vi "Main.vi"() -> ()   [LabVIEW 2019]
panel:
  in  "Warning sound":bool
  in  "Bypass the FMag status":bool
  out "Beam Permit":bool
  in  "Force ON Beam permit":bool
  in  "Force OFF Beam permit":bool
  out "Beam permit status":string
  out "Warning play time":u32
  out "TCP":bool
  in  "Exit VI":bool
  out "Fmag Low Current attemps":i32
  out "Error status":T1(ring)
  out "FMag monitor":u8(slide) scale=0.0..25.0
  out "chart_temp 2":waveform(dbl)[](graph)=[{"t0"=timestamp(3772890114.31303 s since 1904-01-01), "dt"=1.0, "Y"=[0.8687935985565186]}, {"t0"=timestamp(3772890114.31303 s since 1904-01-01), "dt"=1.0, "Y"=[86.87935985565186]}, {"t0"=timestamp(3772890114.31303 s since 1904-01-01), "dt"=1.0, "Y"=[30.48853325313992]}, {"t0"=timestamp(3772890114.31303 s since 1904-01-01), "dt"=1.0, "Y"=[303.6385332531399]}] caption="FMag Current"
  out "FMag Current (A)":dbl
  out "error out":errorcluster
  out "Target  Ready":bool
  out "FMag Ready":bool
  # "SpinQuest Beam Permit Signaller"
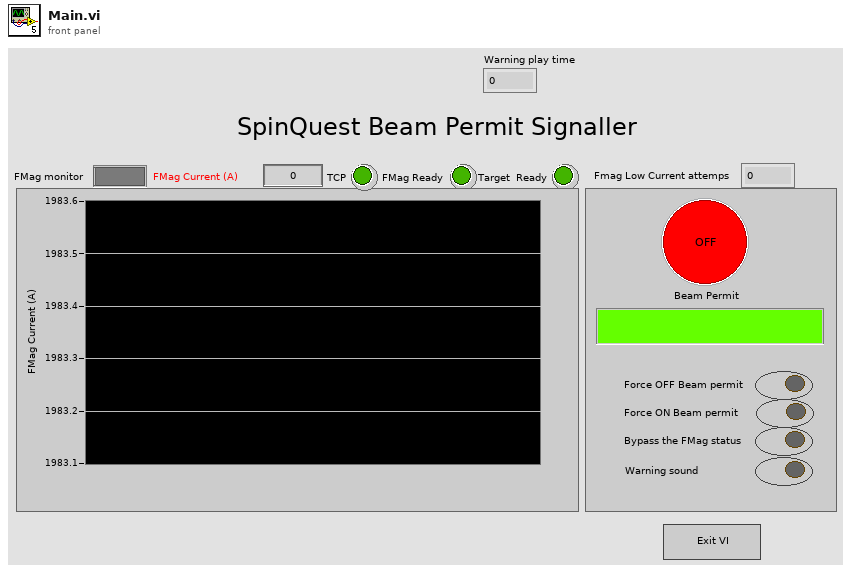
[diagram p1: front panel]
types:
  T1 = enum16{"No Error", "Les than 1800", "Les than 1500", "Les than 200", "Read out Error"}
  T2 = typedef "Sound Output Task ID.ctl" = u32
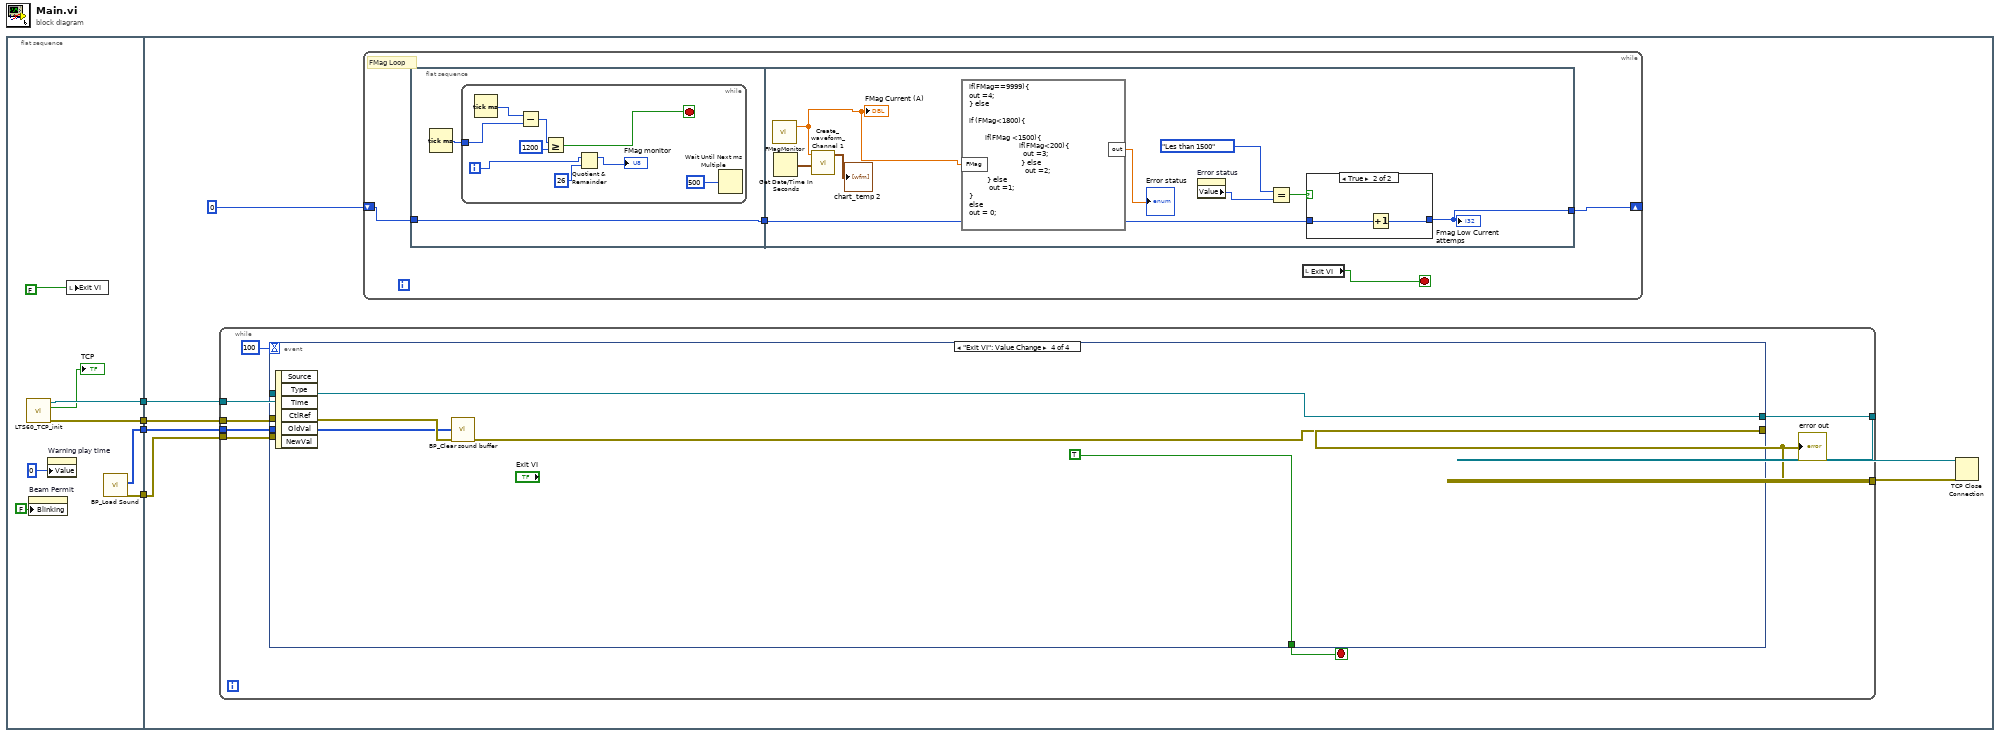
[diagram p0: block diagram]
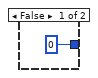
[diagram p2: hidden frame]
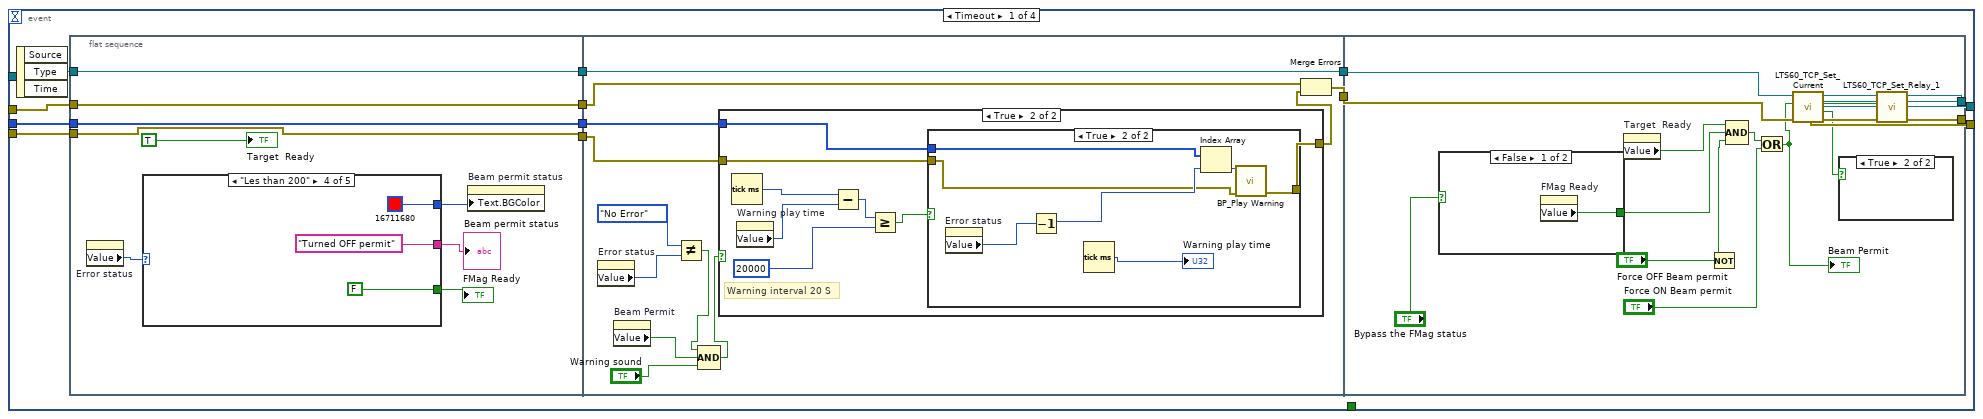
[diagram p3: hidden frame]
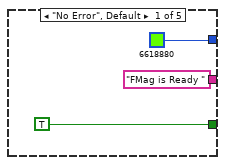
[diagram p4: hidden frame]
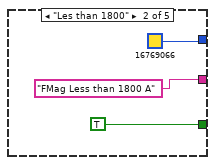
[diagram p5: hidden frame]
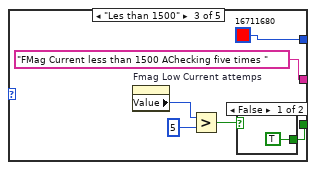
[diagram p6: hidden frame]
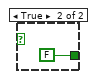
[diagram p7: hidden frame]
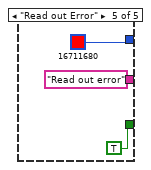
[diagram p8: hidden frame]
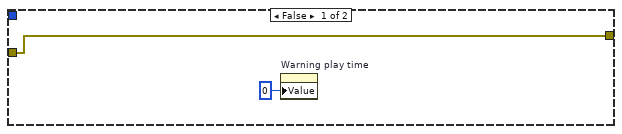
[diagram p9: hidden frame]
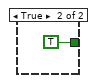
[diagram p12: hidden frame]
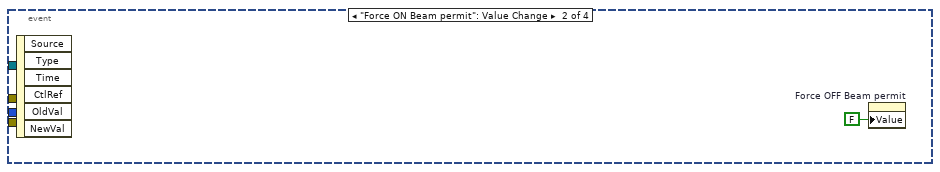
[diagram p13: hidden frame]
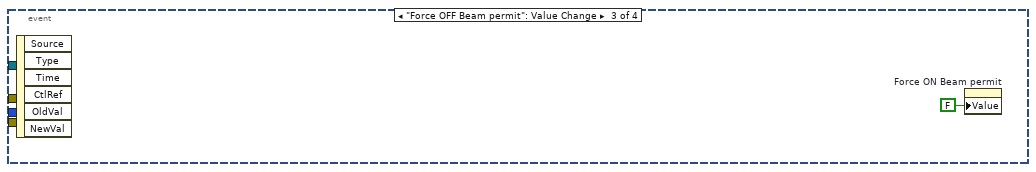
[diagram p14: hidden frame]
diagram:
  n1 = flat-sequence {
    tunnel: [w12] -> w4
    tunnel: [w11] -> w3
    tunnel: [w7] -> w2
    tunnel: [w5] -> w1
    tunnel: w4 -> [w14]
    tunnel: w3 -> [w17]
    tunnel: w2 -> [w15]
    tunnel: w1 -> [w13]
    frame #0 {
      n2 = call "LTS60_TCP_init.vi"() -> ("error out"=w12:errorcluster, "TCP Connected"=→"TCP":bool, "connection ID out"=w11:refnum<k5>)  [unwired: 9 in]
      n3 = property on="Beam Permit" class="Bool (strict)"("Blinking"=FALSE) -> ()  [unwired: 2 in, 2 out]
      n4 = property on="Warning play time" class="DigNum (strict)"("Value"=u32 0 ("Warning play time")) -> ()  [unwired: 2 in, 2 out]
      n5 = local write "Exit VI"(FALSE ("Exit VI")) -> ()
      n6 = call "BP_Load Sound.vi"() -> ("error out"=w5:errorcluster, "Sound Array"=w7:T2[])  [unwired: 9 in, 1 out]
    }
    frame #1 {
      n7 = while {
        tunnel: [w52] -> w18
        tunnel: [w51] -> w19
        tunnel: w14 -> [w50]
        tunnel: w17 -> [w49]
        tunnel: w15 -> [w48]
        tunnel: w13 -> [w47]
        stop <- w54 stop-if-true
        n8 = event shown="[3] \"Exit VI\": Value Change" {
          selector: _ -> [_ _ _ _]
          dyn-events: _ -> [_ _ _ _]
          timeout: 100 -> [_ _ _ _]
          tunnel: [_ _ _ TRUE] -> w54
          tunnel: [w66 _ _ w146] -> w52
          tunnel: [w65 _ _ w149] -> w51
          tunnel: w49 -> [w63 _ _ w149]
          tunnel: w50 -> [w60 _ _ w148]
          tunnel: w48 -> [w58 _ _ w147]
          tunnel: w47 -> [w55 _ _ _]
          event Timeout {
            n9 = event-data() -> ()  [unwired: 1 in, 3 out]
            n10 = flat-sequence {
              tunnel: [w74] -> w64
              tunnel: w63 -> [w74]
              tunnel: [w73] -> w61
              tunnel: w60 -> [w73]
              tunnel: w58 -> [w69]
              tunnel: [w69] -> w57
              tunnel: [w68] -> w56
              tunnel: w55 -> [w68]
              tunnel: w64 -> [w107]
              tunnel: [w107] -> w62
              tunnel: w61 -> [w96]
              tunnel: [w98] -> w59
              tunnel: w57 -> [w104]
              tunnel: w56 -> [w99]
              tunnel: [w137] -> w66
              tunnel: [w136] -> w65
              tunnel: w62 -> [w140]
              tunnel: w59 -> [w134]
              frame #0 {
                n11 = property on="Error status" class="Enum (strict)"() -> ("Value"=w70:T1)  [unwired: 2 in, 2 out]
                n12 = case shown="\"Les than 200\"" w70 {
                  tunnel: [TRUE ("Magnet status") TRUE ("Magnet status") w87 FALSE ("Magnet status") TRUE ("Magnet status")] -> w71
                  tunnel: ["FMag is Ready " ("Beam permit status") "FMag Less than 1800 A" ("Beam permit status") "FMag Current less than 1500 AChecking five times " ("Beam permit status") "Turned OFF permit" ("Beam permit status") "Read out error" ("Beam permit status")] -> w72
                  tunnel: [u32 6618880 ("Text.Text Colors:BG Color") u32 16769066 ("Text.Text Colors:BG Color") u32 16711680 ("Text.Text Colors:BG Color") u32 16711680 ("Text.Text Colors:BG Color") u32 16711680 ("Text.Text Colors:BG Color")] -> w67
                  frame "No Error", Default {
                  }
                  frame "Les than 1800" {
                  }
                  frame "Les than 1500" {
                    n13 = property on="Fmag Low Current attemps" class="DigNum (strict)"() -> ("Value"=w86:i32)  [unwired: 2 in, 2 out]
                    n14 = Greater?(x=w86, y=5) -> (0:w84:bool)
                    n15 = case shown="False" w84 {
                      tunnel: [TRUE ("Magnet status") FALSE ("Magnet status")] -> w87
                      frame False {
                      }
                      frame True {
                      }
                    }
                  }
                  frame "Les than 200" {
                  }
                  frame "Read out Error" {
                  }
                }
                "FMag Ready" <- w71
                "Beam permit status" <- w72
                n16 = property on="Beam permit status" class="Str"("Text.BGColor"=w67) -> ()  [unwired: 2 in, 2 out]
                "Target  Ready" <- TRUE ("Target  status")
              }
              frame #1 {
                n17 = property on="Error status" class="Enum (strict)"() -> ("Value"=w106:T1)  [unwired: 2 in, 2 out]
                n18 = property on="Beam Permit" class="Bool (strict)"() -> ("Value"=w102:bool)  [unwired: 2 in, 2 out]
                n19 = Not Equal?(x=T1."No Error", y=w106) -> (x != y?=w101:bool)
                n20 = Compound Arithmetic op=AND(w101, w102, "Warning sound") -> (w100:bool)
                n21 = case shown="True" w100 {
                  tunnel: w104 -> [_ w112]
                  tunnel: [w108 w111] -> w97
                  tunnel: w99 -> [w108 w110]
                  frame False {
                    n22 = property on="Warning play time" class="DigNum (strict)"("Value"=u32 0 ("Warning play time")) -> ()  [unwired: 2 in, 2 out]
                  }
                  frame True {
                    # "Warning interval 20 S"
                    n23 = Tick Count (ms)() -> (millisecond timer value=w117:u32)
                    n24 = property on="Warning play time" class="DigNum (strict)"() -> ("Value"=w116:u32)  [unwired: 2 in, 2 out]
                    n25 = Subtract(x=w117, y=w116) -> (x-y=w115:u32)
                    n26 = Greater Or Equal?(x=w115, y=u32 20000) -> (x >= y?=w113:bool)
                    n27 = case shown="True" w113 {
                      tunnel: w112 -> [_ w123]
                      tunnel: [w118 w120] -> w111
                      tunnel: w110 -> [w118 w119]
                      frame False {
                      }
                      frame True {
                        n28 = property on="Error status" class="Enum (strict)"() -> ("Value"=w125:T1)  [unwired: 2 in, 2 out]
                        n29 = Decrement(x=w125) -> (x-1=w122:T1)
                        n30 = Tick Count (ms)() -> (millisecond timer value=→"Warning play time":u32)
                        n31 = Index Array(array=w123, index=w122) -> (element=w121:T2)
                        n32 = call "BP_Play Warning.vi"("error in (no error)"=w119, "task ID"=w121) -> ("error out"=w120:errorcluster)  [unwired: 8 in, 1 out]
                      }
                    }
                  }
                }
                n33 = Merge Errors(w96, w97) -> (w98:errorcluster)
              }
              frame #2 {
                n34 = case shown="False" "Bypass the FMag status" {
                  tunnel: [w142 TRUE ("Value")] -> w130
                  frame False {
                    n35 = property on="FMag Ready" class="Bool (strict)"() -> ("Value"=w142:bool)  [unwired: 2 in, 2 out]
                  }
                  frame True {
                  }
                }
                n36 = property on="Target  Ready" class="Bool (strict)"() -> ("Value"=w141:bool)  [unwired: 2 in, 2 out]
                n37 = Not(x="Force OFF Beam permit") -> (.not. x?=w129:bool)
                n38 = Compound Arithmetic op=AND(w141, w130, w129) -> (w132:bool)
                n39 = Or(x=w132, y="Force ON Beam permit") -> (x .or. y?=w127:bool)
                "Beam Permit" <- w127
                n40 = call "LTS60_TCP_Set_Current.vi"("error in (no error)"=w134, "Beam"=w127, "connection ID"=w140) -> ("error out"=w138:errorcluster, "Acknowladged"=w126:bool, "Beam out"=w135:bool, "connection ID out"=w139:refnum<k5>)  [unwired: 5 in]
                n41 = case shown="True" w126 {
                  frame False {
                  }
                  frame True {
                  }
                }
                n42 = call "LTS60_TCP_Set_Relay_1.vi"("error in (no error)"=w138, "Beam"=w135, "connection ID"=w139) -> ("error out"=w137:errorcluster, "connection ID out"=w136:refnum<k5>)  [unwired: 6 in, 1 out]
              }
            }
          }
          event "Force ON Beam permit": Value Change {
            n43 = event-data() -> ()  [unwired: 1 in, 6 out]
            n44 = property on="Force OFF Beam permit" class="Bool (strict)"("Value"=FALSE ("Force OFF Beam permit")) -> ()  [unwired: 2 in, 2 out]
          }
          event "Force OFF Beam permit": Value Change {
            n45 = event-data() -> ()  [unwired: 1 in, 6 out]
            n46 = property on="Force ON Beam permit" class="Bool (strict)"("Value"=FALSE ("Force ON Beam permit")) -> ()  [unwired: 2 in, 2 out]
          }
          event "Exit VI": Value Change {
            n47 = event-data() -> ()  [unwired: 1 in, 6 out]
            n48 = call "BP_Clear sound buffer.vi"("error in (no error)"=w148, "array"=w147) -> ("error out"=w146:errorcluster)  [unwired: 9 in]
          }
        }
        "error out" <- w52
      }
      n49 = while {
        shift-right: [w21] -> _
        shift-left: 0 ("Low Fmag attemps") -> [w23]
        stop <- w20 stop-if-true
        # "FMag Loop"
        n50 = flat-sequence {
          tunnel: w23 -> [w24]
          tunnel: [w24] -> w22
          tunnel: w22 -> [w39]
          tunnel: [w38] -> w21
          frame #0 {
            n51 = Tick Count (ms)() -> (millisecond timer value=w25:u32)
            n52 = while {
              tunnel: w25 -> [w32]
              i -> [w26]
              stop <- w31 stop-if-true
              n53 = Tick Count (ms)() -> (millisecond timer value=w33:u32)
              n54 = Subtract(x=w33, y=w32) -> (x-y=w30:u32)
              n55 = Greater Or Equal?(x=w30, y=u32 1200) -> (x >= y?=w31:bool)
              n56 = Quotient & Remainder(x=w26, y=u32 26) -> (x-y*floor(x/y)=→"FMag monitor":u32)  [unwired: 1 out]
              n57 = Wait Until Next ms Multiple(millisecond multiple=u32 500) -> ()  [unwired: 1 out]
            }
          }
          frame #1 {
            n58 = call "FMagMonitor.vi"() -> ("FMag Current"=w35:dbl)  [unwired: 2 in, 1 out]
            "FMag Current (A)" <- w35
            n59 = Get Date/Time In Seconds() -> (seconds since 1Jan1904=w43:timestamp)
            n60 = call "Create_waveform_Channel 1.vi"("time"=w43, "Channel 1"=w35) -> ("waveform_array"=→"chart_temp 2":waveform(dbl)[])  [unwired: 9 in]
            n61 = formula code="if(FMag==9999){\nout =4;\n} else\n\nif (FMag<1800){\n       \n        if(FMag <1500){\n                         if(FMag<200){\n                           out =3;\n                          } else \n                            out =2;\n         } else\n          out =1;\n}\nelse\nout = 0;"("FMag"=w35) -> ("out"=→"Error status":dbl)
            n62 = property on="Error status" class="Enum (strict)"() -> ("Value"=w37:T1)  [unwired: 2 in, 2 out]
            n63 = Equal?(x=T1."Les than 1500", y=w37) -> (x = y?=w40:bool)
            n64 = case shown="True" w40 {
              tunnel: [0 ("Low Fmag attemps") w46] -> w38
              tunnel: w39 -> [_ w45]
              frame False {
              }
              frame True {
                n65 = Increment(x=w45) -> (x+1=w46:i32)
              }
            }
            "Fmag Low Current attemps" <- w38
          }
        }
        n66 = local read "Exit VI"() -> (w20:bool)
      }
      n67 = TCP Close Connection(connection ID=w19, error in (no error)=w18) -> ()  [unwired: 1 in, 2 out]
    }
  }
